vi "Process Incoming Frames.vi"(0 "Variables In":T1={"Process Ref"=refnum, "Comm Ref"=refnum, "Data Refs"={"ProtectionsAndCounters.Ref"=refnum, "Signals.Ref"=refnum, "Status.Ref"=refnum, "Overrides"=refnum, "IncomingSignals.Ref"=refnum, "CtrandProtctnVld.Ref"=refnum, "RcvTime.Ref"=refnum, "TimeDiff.Ref"=refnum, "IncomingProtCtr.Ref"=refnum}, "Settings"={"Name"="", "Priority"=0, "XNET Settings"={"Database"="", "Cluster"="", "Port"="", "Baud rate [Bd]"=0, "Termination"=0, "CAN I/O Mode"=0, "FD Baud rate [Bd]"=500000, "Priority"=100, "Use Legacy"=FALSE, "FD ISO Mode"=0}, "FPGA Session"=0, "Outgoing CAN Session"="", "Outgoing Frame Count"=0, "Outgoing Frames"=[], "Incoming CAN Session"="", "Incoming Frame Count"=0, "Incoming Frames"=[], "Incoming Values"={"Signal Values"=[], "Signal Invalid Values"=[], "ProtCtr Sig Values"=[], "Timestamps"=[], "Time Differences"=[], "IDs"=[]}}, "Stream Refs"={"Addon"="", "Port"="", "Filter Ref"=refnum, "Default Filter"={"ID Filters"=[], "Direction Filter"=enum."Tx/Rx", "Type Filter"=enum."All"}, "Port Settings"={"Mode"=0, "Baud Rate"=0, "Termination"=0, "FD ISO Mode"=0, "FD Baud Rate"=0}}} {"Stream Refs"."Port Settings"."FD ISO Mode" items=["ISO", "Non ISO", "ISO Legacy"]; "Stream Refs"."Port Settings"."Termination" items=["Off", "On"]; "Stream Refs"."Port Settings"."Mode" items=["CAN 2.0", "CAN FD", "CAN FD+BRS"]; "Settings"."XNET Settings"."FD ISO Mode" items=["ISO", "Non ISO", "ISO Legacy"]; "Settings"."XNET Settings"."CAN I/O Mode" items=["CAN 2.0", "CAN FD", "CAN FD+BRS"]; "Settings"."XNET Settings"."Termination" items=["Off", "On"]}, 11 "error in":errorcluster) -> (4 "Variables Out":T1={"Process Ref"=refnum, "Comm Ref"=refnum, "Data Refs"={"ProtectionsAndCounters.Ref"=refnum, "Signals.Ref"=refnum, "Status.Ref"=refnum, "Overrides"=refnum, "IncomingSignals.Ref"=refnum, "CtrandProtctnVld.Ref"=refnum, "RcvTime.Ref"=refnum, "TimeDiff.Ref"=refnum, "IncomingProtCtr.Ref"=refnum}, "Settings"={"Name"="", "Priority"=0, "XNET Settings"={"Database"="", "Cluster"="", "Port"="", "Baud rate [Bd]"=0, "Termination"=0, "CAN I/O Mode"=0, "FD Baud rate [Bd]"=500000, "Priority"=100, "Use Legacy"=FALSE, "FD ISO Mode"=0}, "FPGA Session"=0, "Outgoing CAN Session"="", "Outgoing Frame Count"=0, "Outgoing Frames"=[], "Incoming CAN Session"="", "Incoming Frame Count"=0, "Incoming Frames"=[], "Incoming Values"={"Signal Values"=[], "Signal Invalid Values"=[], "ProtCtr Sig Values"=[], "Timestamps"=[], "Time Differences"=[], "IDs"=[]}}, "Stream Refs"={"Addon"="", "Port"="", "Filter Ref"=refnum, "Default Filter"={"ID Filters"=[], "Direction Filter"=enum."Tx/Rx", "Type Filter"=enum."All"}, "Port Settings"={"Mode"=0, "Baud Rate"=0, "Termination"=0, "FD ISO Mode"=0, "FD Baud Rate"=0}}} {"Stream Refs"."Port Settings"."FD ISO Mode" items=["ISO", "Non ISO", "ISO Legacy"]; "Stream Refs"."Port Settings"."Termination" items=["Off", "On"]; "Stream Refs"."Port Settings"."Mode" items=["CAN 2.0", "CAN FD", "CAN FD+BRS"]; "Settings"."XNET Settings"."FD ISO Mode" items=["ISO", "Non ISO", "ISO Legacy"]; "Settings"."XNET Settings"."CAN I/O Mode" items=["CAN 2.0", "CAN FD", "CAN FD+BRS"]; "Settings"."XNET Settings"."Termination" items=["Off", "On"]}, 15 "error out":errorcluster)   [LabVIEW 2019, in "Ghost Bus Addon Engine.lvlib"]
doc: "This example demonstrates receiving automatically converted values of signals, along with the associated timestamp value, using an NI-XNET Signal Input XY session. \n\nThis example can run against the CAN Signal Output XY example, assuming you have a properly terminated CAN cable connected to two CAN ports.\n\nIf you have no database aliases on your system, the example automatically loads the nixnet_example database."
uses:
  Ghost Bus Addon Engine.lvlib
  Types/RT Async Engine Variables.ctl
  <vilib>/NI/NIVS Inline Async API/_VS Inline Async API/Process/Process.lvclass
  <vilib>/NI/NI VeriStand Addon Network Comm/Engine/VeriStand Comm.lvclass
  Types/RT Data References.ctl
  <vilib>/NI/NIVS Inline Async API/_Data Access Engine/Data Access Engine/Types/Write.DVR.ctl
  <vilib>/NI/NIVS Inline Async API/_Data Access Engine/Access Type Classes/Write/Write.lvclass
  <vilib>/NI/NIVS Inline Async API/_Data Access Engine/Data Access Engine/Types/Read.DVR.ctl
  <vilib>/NI/NIVS Inline Async API/_Data Access Engine/Access Type Classes/Read/Read.lvclass
  Types/RT Async Engine Settings.ctl
  Addon Shared/Types/XNET Settings.ctl
  SubModules/Frame-Protection-Support/Source/Engine/Types/RT Frame Settings.ctl
  SubModules/Frame-Protection-Support/Source/Shared/Types/Exported Frame Type.ctl
  SubModules/Frame-Protection-Support/Source/Engine/Types/RT Protection Configuration.ctl
  SubModules/Frame-Protection-Support/Source/Shared/Types/Protection Type.ctl
  SubModules/Frame-Protection-Support/Source/Shared/Types/XNET Signal Configuration.ctl
  SubModules/Frame-Protection-Support/Source/Shared/Types/Exported Counter Settings.ctl
  SubModules/Frame-Protection-Support/Source/Shared/Types/Exported Event Trigger Type.ctl
  SubModules/Frame-Protection-Support/Source/Engine/Types/RT Frame Incoming Values.ctl
  SubModules/CAN-Streaming-Support/Source/Addon/Addon Engine/Types/Engine Stream Refs.ctl
  SubModules/CAN-Streaming-Support/Source/Addon/Addon Shared/Types/Direction Filter.ctl
  SubModules/CAN-Streaming-Support/Source/Addon/Addon Shared/Types/Type Filter.ctl
  SubModules/CAN-Streaming-Support/Source/Addon/Addon Shared/Types/Filter Parameters.ctl
  SubModules/CAN-Streaming-Support/Source/Addon/Addon Engine/Types/Engine Stream Port Settings.ctl
  <vilib>/NI/NIVS Inline Async API/_Data Access Engine/Access Type Classes/Write/Write.lvclass/Write.ctl
  SubModules/Frame-Protection-Support/Source/Engine/SubVIs/Get Frame Time Info.vi
  SubModules/Frame-Protection-Support/Source/Engine/SubVIs/Process Regular Signal.vi
  SubModules/Frame-Protection-Support/Source/Engine/SubVIs/Process Counter Signals.vi
  SubModules/Frame-Protection-Support/Source/Engine/SubVIs/Process Protection Signals.vi
  <vilib>/NI/NIVS Inline Async API/_Data Access Engine/Data Access Engine/Methods/Data.Processes.Execute.vi
  <vilib>/NI/NIVS Inline Async API/_Data Access Engine/Data Access Engine/Methods/Write.Data.vi
  SubModules/Frame-Protection-Support/Source/Engine/SubVIs/Calculate Protection Value.vi
  <vilib>/NI/NIVS Inline Async API/_Data Access Engine/Access Type Classes/Write/Write.ProcessData.vi
  SubModules/Frame-Protection-Support/Source/Engine/SubVIs/Get Protection Signals.vi
  <vilib>/NI/NIVS Inline Async API/_Data Access Engine/Access Type Classes/Write/Write.Buffer.vi
  <vilib>/NI/NIVS Inline Async API/_Data Access Engine/Access Type Classes/Write/Write.Commit.vi
  <vilib>/xnet/xnet.llb/XNET Read (Frame CAN).vi
  <vilib>/xnet/xnet.llb/XNET Convert.vi
  <vilib>/xnet/xnet.llb/XNET Convert (Frame CAN to Signal).vi
  <vilib>/xnet/xnet.llb/XNET Convert (Signal to Frame Raw).vi
  SubModules/Frame-Protection-Support/Source/Engine/Protection and Counter Support Engine.lvlib
  <vilib>/NI/NIVS Inline Async API/_Data Access Engine/Data Access Engine/Data Access Engine.lvclass
  SubModules/Frame-Protection-Support/Source/Shared/Protection and Counter Support Shared.lvlib
  Addon Shared/Ghost Bus Addon Shared.lvlib
  SubModules/CAN-Streaming-Support/Source/Addon/Addon Shared/CAN Stream Support Shared.lvlib
  SubModules/CAN-Streaming-Support/Source/Addon/Addon Engine/CAN Stream Support Engine.lvlib
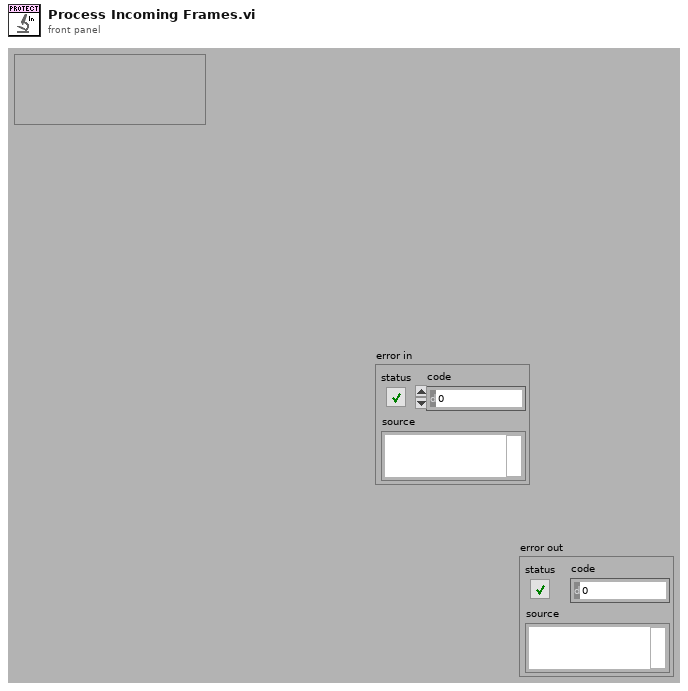
[diagram p1: front panel]
types:
  T1 = typedef "Ghost Bus Addon Engine.lvlib/RT Async Engine Variables.ctl" = cluster{"Process Ref":refnum<class "Process.lvclass">, "Comm Ref":refnum<class "VeriStand Comm.lvclass">, "Data Refs":T2, "Settings":T5, "Stream Refs":T15}
  T2 = typedef "Ghost Bus Addon Engine.lvlib/RT Data References.ctl" = cluster{"ProtectionsAndCounters.Ref":T3, "Signals.Ref":T4, "Status.Ref":T3, "Overrides":T4, "IncomingSignals.Ref":T3, "CtrandProtctnVld.Ref":T3, "RcvTime.Ref":T3, "TimeDiff.Ref":T3, "IncomingProtCtr.Ref":T3}
  T3 = typedef "Data Access Engine.lvlib/Data Access Engine.lvclass/Write.DVR.ctl" = refnum<data-value>
  T4 = typedef "Data Access Engine.lvlib/Data Access Engine.lvclass/Read.DVR.ctl" = refnum<data-value>
  T5 = typedef "Ghost Bus Addon Engine.lvlib/RT Async Engine Settings.ctl" = cluster{"Name":string, "Priority":i32, "XNET Settings":T6, "FPGA Session":u32, "Outgoing CAN Session":refnum<k21>, "Outgoing Frame Count":i32, "Outgoing Frames":T7[], "Incoming CAN Session":refnum<k21>, "Incoming Frame Count":i32, "Incoming Frames":T7[], "Incoming Values":T14}
  T6 = typedef "Ghost Bus Addon Shared.lvlib/XNET Settings.ctl" = cluster{"Database":refnum<k21>, "Cluster":refnum<k21>, "Port":string, "Baud rate [Bd]":u64, "Termination":u32, "CAN I/O Mode":u32, "FD Baud rate [Bd]":u64, "Priority":i32, "Use Legacy":bool, "FD ISO Mode":u32}
  T7 = typedef "Protection and Counter Support Engine.lvlib/RT Frame Settings.ctl" = cluster{"Type":T8, "Frame ID":u32, "Payload Length":u32, "VS Offset":i32, "VS Length":i32, "Frame Conversion":refnum<k21>, "Frame.Data":dbl[], "Generation Period":u32, "Time Since Last Generation":u32, "Generation Iterations":u32, "Generation Counter":u32, "Has Protection?":bool, "Protection Configurations":T9[], "Has Counter?":bool, "Counter Configurations":T12[], "Has Disable?":bool, "Disable VS Index":i32, "Transmit Trigger":T13, "Trigger VS Index":i32}
  T8 = typedef "Protection and Counter Support Shared.lvlib/Exported Frame Type.ctl" = enum16{"Periodic", "Event", "Periodic/Event"}
  T9 = typedef "Protection and Counter Support Engine.lvlib/RT Protection Configuration.ctl" = cluster{"Protection Frame Index":i32, "Protection Type":T10, "Data Indeces":i32[], "Data Array":dbl[], "Check Sum Conversion":refnum<k21>, "CRC Channels":T11[], "Protection VS Index":i32, "Counter Data Index":i32, "Override Index":i32, "Override Value Index":i32}
  T10 = typedef "Protection and Counter Support Shared.lvlib/Protection Type.ctl" = enum16{"Arb ID + Bytes Checksum with Inversion", "Arb ID + Bytes CRC with Inversion", "Reversed Raw Signal Checksum with Inversion", "Concatenated Two's Compliment"}
  T11 = typedef "Protection and Counter Support Shared.lvlib/XNET Signal Configuration.ctl" = cluster{"Start Bit":i32, "Name":string, "Number of bits":i32, "Scale":dbl, "Offset":dbl, "Data Type":u32, "Counter":bool}
  T12 = typedef "Protection and Counter Support Shared.lvlib/Exported Counter Settings.ctl" = cluster{"Frame Index":i32, "Max Count":dbl, "VS Index":i32, "Bit Length":i64, "Override Index":i32, "Override Value Index":i32}
  T13 = typedef "Protection and Counter Support Shared.lvlib/Exported Event Trigger Type.ctl" = enum16{"Channel value change", "Trigger channel (not zero)", "Channel value change or trigger channel (not zero)", "Trigger channel (any value change)", "Channel value change or trigger channel (any value change)"}
  T14 = typedef "Protection and Counter Support Engine.lvlib/RT Frame Incoming Values.ctl" = cluster{"Signal Values":dbl[], "Signal Invalid Values":dbl[], "ProtCtr Sig Values":dbl[], "Timestamps":timestamp[], "Time Differences":dbl[], "IDs":u32[]}
  T15 = typedef "CAN Stream Support Engine.lvlib/Engine Stream Refs.ctl" = cluster{"Addon":string, "Port":refnum<k21>, "Filter Ref":refnum<data-value>, "Default Filter":T16, "Port Settings":T19}
  T16 = typedef "CAN Stream Support Shared.lvlib/Filter Parameters.ctl" = cluster{"ID Filters":u32[], "Direction Filter":T17, "Type Filter":T18}
  T17 = typedef "CAN Stream Support Shared.lvlib/Direction Filter.ctl" = enum16{"Tx/Rx", "Rx", "Tx"}
  T18 = typedef "CAN Stream Support Shared.lvlib/Type Filter.ctl" = enum16{"All", "CAN Data", "CAN Remote", "CAN Bus Error", "CAN 2.0 Data", "CAN FD Data", "CAN FD+BRS Data", "J1939 Data", "Delay", "Log Trigger", "Start Trigger"}
  T19 = typedef "CAN Stream Support Engine.lvlib/Engine Stream Port Settings.ctl" = cluster{"Mode":u32, "Baud Rate":u64, "Termination":u32, "FD ISO Mode":u32, "FD Baud Rate":u64}
  T20 = typedef "XNET Frame CAN.ctl" = cluster{"timestamp":timestamp, "payload":u8[], "identifier":u32, "type":T21, "extended?":bool, "echo?":bool}
  T21 = typedef "XNET Frame Type CAN.ctl" = u8
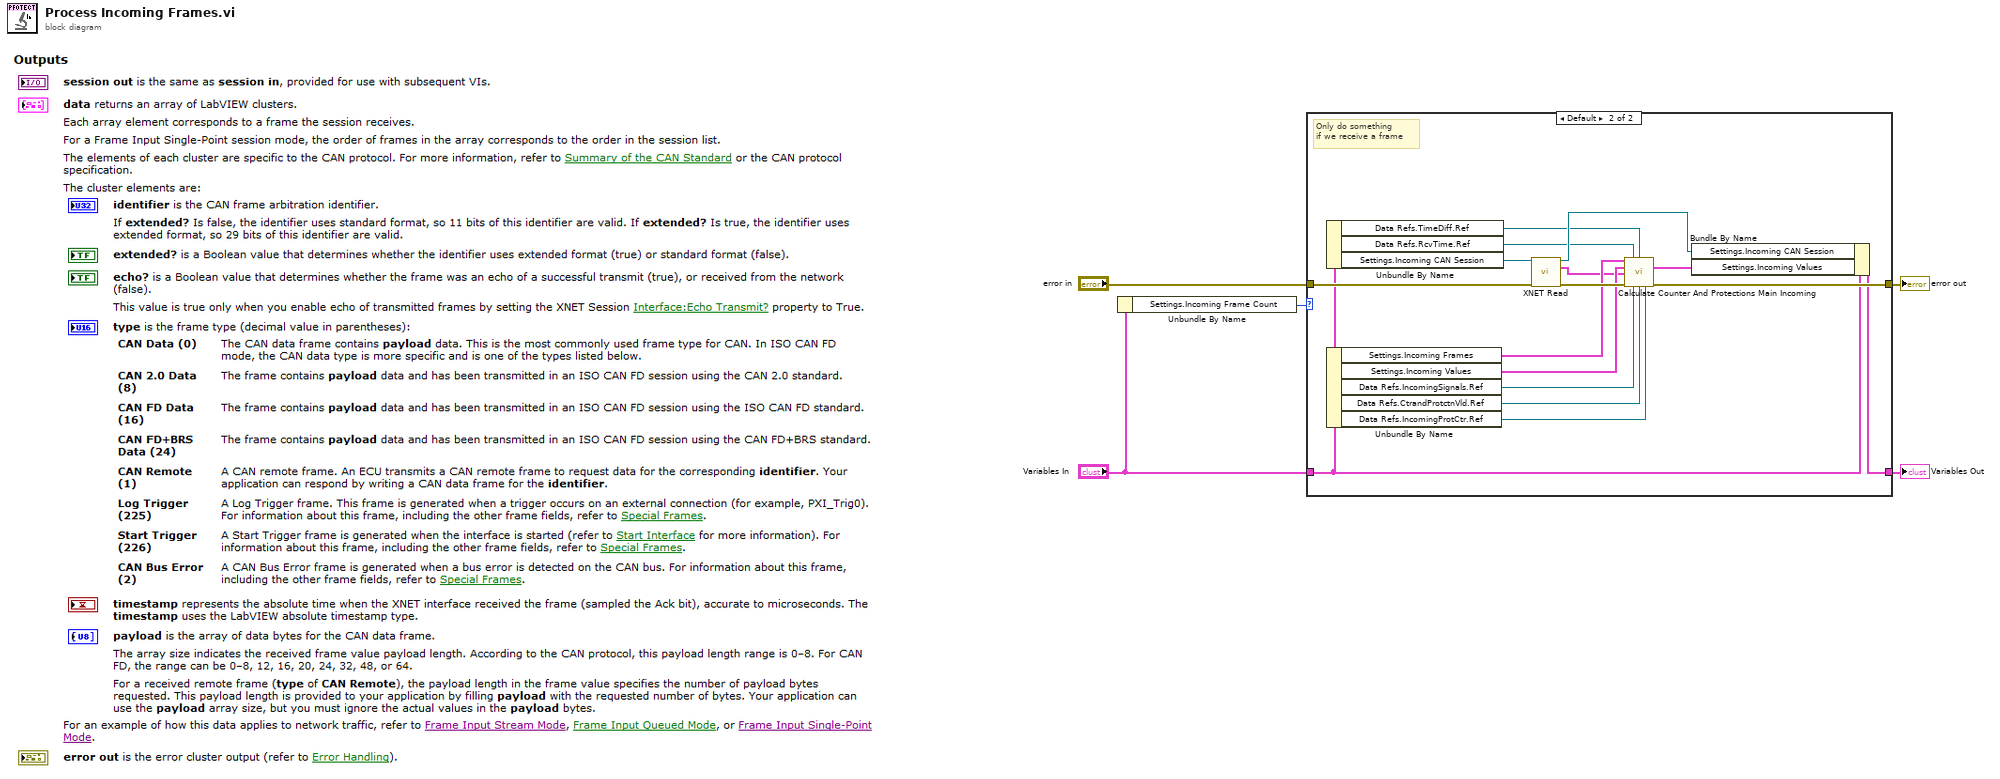
[diagram p0: block diagram]
diagram:
  n1 = Unbundle By Name("Variables In") -> ("Settings.Incoming Frame Count"=w1:i32)
  n2 = case shown="Default" w1 {
    tunnel: [w7 w23] -> w5
    tunnel: "error in" -> [w7 w22]
    tunnel: [w6 w18] -> w3
    tunnel: "Variables In" -> [w6 w19]
    frame 0 {
    }
    frame Default {
      # "Only do something\nif we receive a frame"
      n3 = Unbundle By Name(w19) -> ("Data Refs.TimeDiff.Ref"=w12:T3, "Data Refs.RcvTime.Ref"=w13:T3, "Settings.Incoming CAN Session"=w20:refnum<k21>)
      n4 = Unbundle By Name(w19) -> ("Settings.Incoming Frames"=w10:T7[], "Settings.Incoming Values"=w9:T14, "Data Refs.IncomingSignals.Ref"=w14:T3, "Data Refs.CtrandProtctnVld.Ref"=w15:T3, "Data Refs.IncomingProtCtr.Ref"=w16:T3)
      n5 = call-poly <vilib>:"XNET Read.vi"("session in"=w20, "error in (no error)"=w22) -> ("session out"=w17:refnum<k21>, "data"=w8:T20[], "error out"=w21:errorcluster)  [unwired: 11 out]
      n6 = call "Calculate Counter And Protections Main Incoming.vi"("Incoming Frames"=w10, "TimeStamp.Ref"=w13, "TimeDiff.Ref"=w12, "Incoming Values in"=w9, "data"=w8, "error in (no error)"=w21, "IncomingSignals.Ref"=w14, "CtrandProtctnVld.Ref"=w15, "IncomingProtCtr.Ref"=w16) -> ("Incoming Values out"=w11:T14, "error out"=w23:errorcluster)  [unwired: 5 in]
      n7 = Bundle By Name(cluster=w19, "Settings.Incoming CAN Session"=w17, "Settings.Incoming Values"=w11) -> (w18:T1)
    }
  }
  "error out" <- w5
  "Variables Out" <- w3
